vi "Main.vi"() -> ()   [LabVIEW 2015]
doc: "Use this template to build a simple state machine design pattern. Each state executes code and determines which state to transition to."
uses:
  controls/State.ctl
  controls/Data.ctl
panel:
  out "Current State":string
  out "Data":cluster{"X":dbl, "Y":dbl}[](graph)
  in  "Reset Settings":bool
  in  "Clear Graph":bool
  in  "Analyze Data":bool
  in  "Acquire Data":bool
  in  "Configure Data":bool
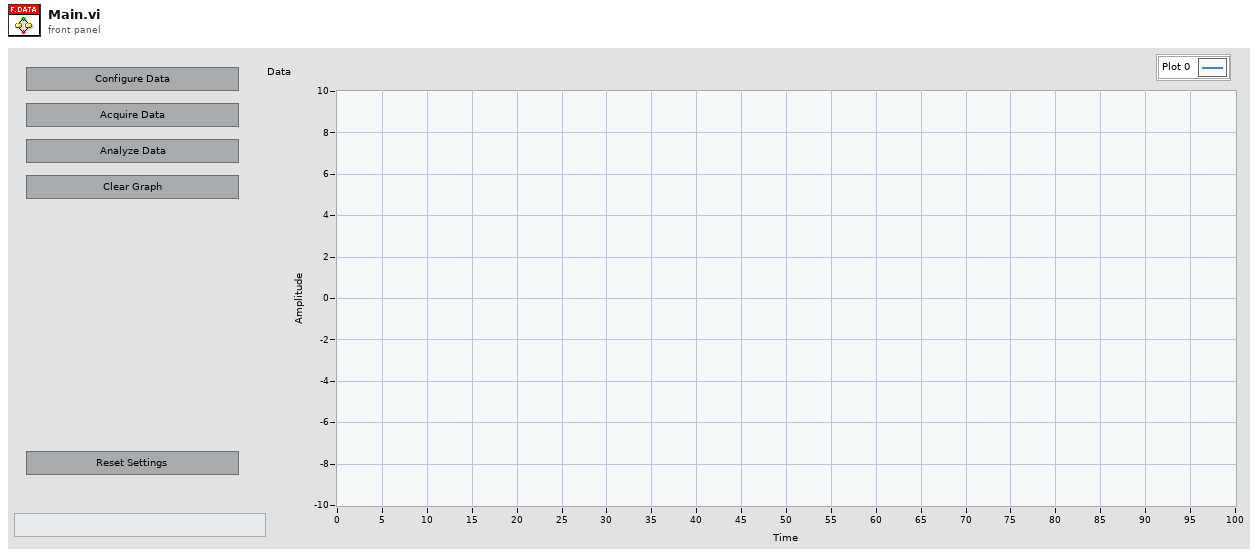
[diagram p1: front panel]
types:
  T1 = typedef "Data.ctl" = cluster{"Boolean <Replace Me>":bool, "String <Replace Me>":string, "Numeric <Replace Me>":dbl}
  T2 = typedef "State.ctl" = enum16{"Initialize", "Wait for Event", "Configure", "Acquire Data", "Update User Interface", "Reset Data", "Clear Data", "Analyse Data", "Stop", "Error"}
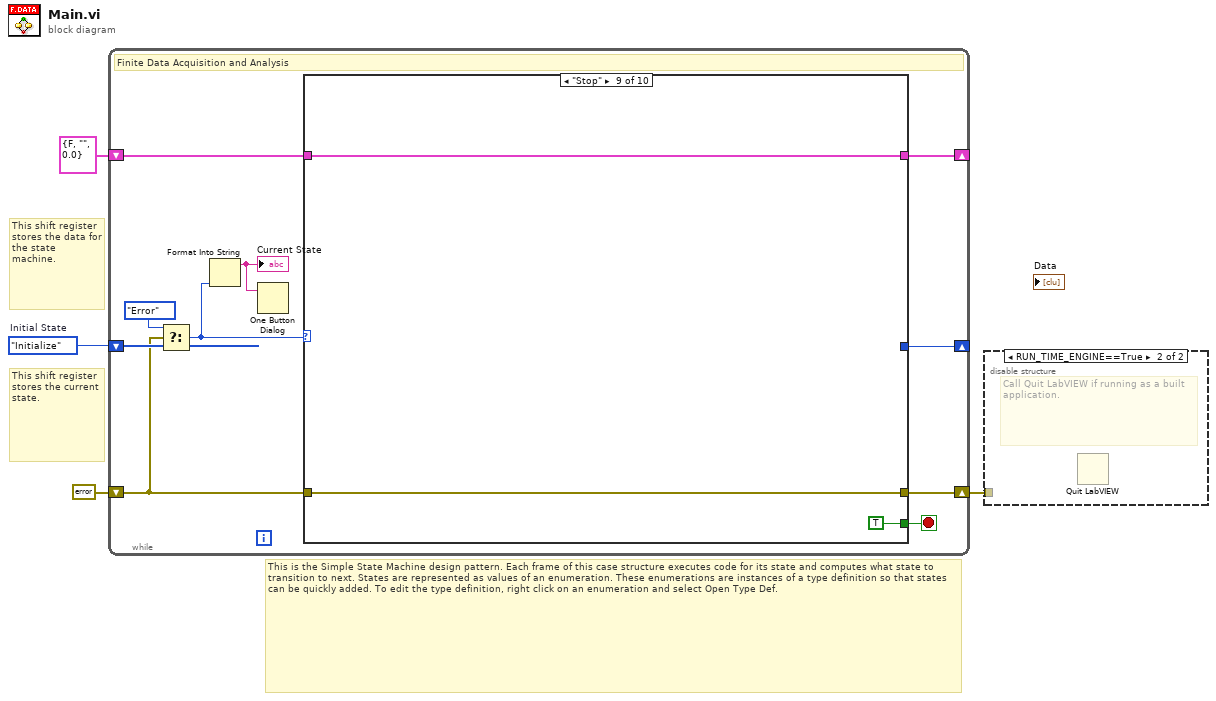
[diagram p0: block diagram]
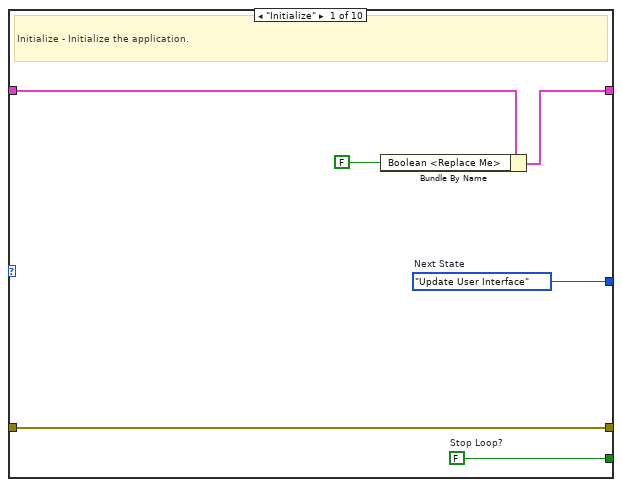
[diagram p3: hidden frame]
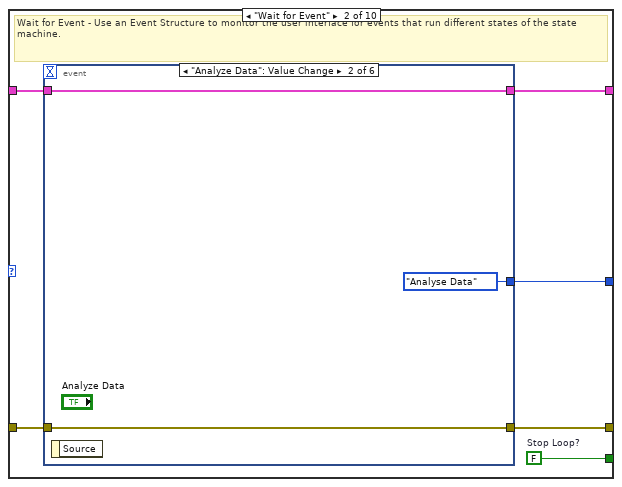
[diagram p4: hidden frame]
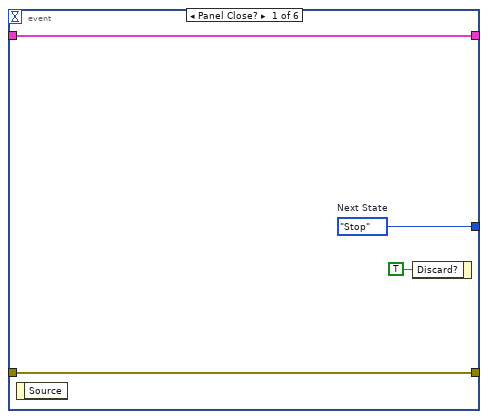
[diagram p5: hidden frame]
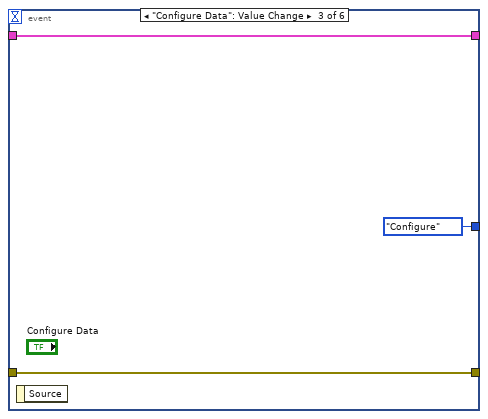
[diagram p6: hidden frame]
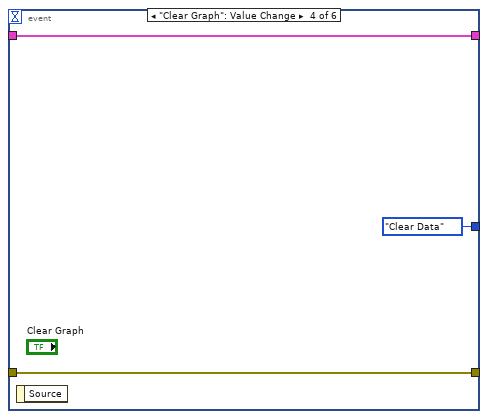
[diagram p7: hidden frame]
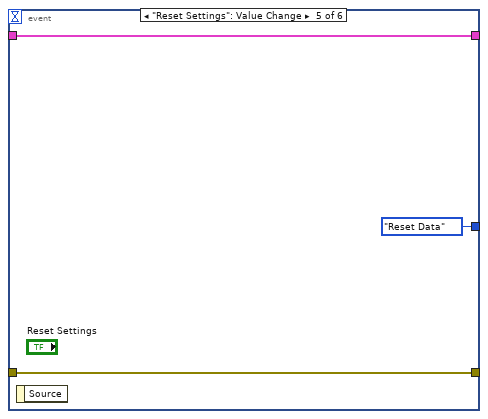
[diagram p8: hidden frame]
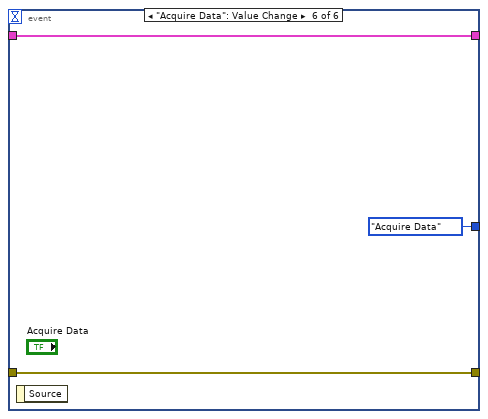
[diagram p9: hidden frame]
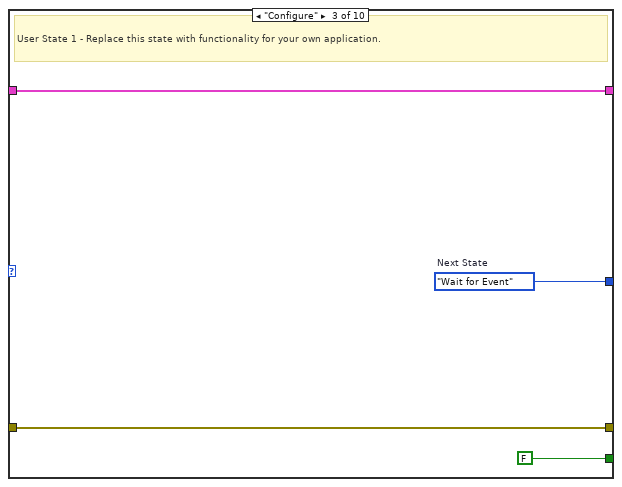
[diagram p10: hidden frame]
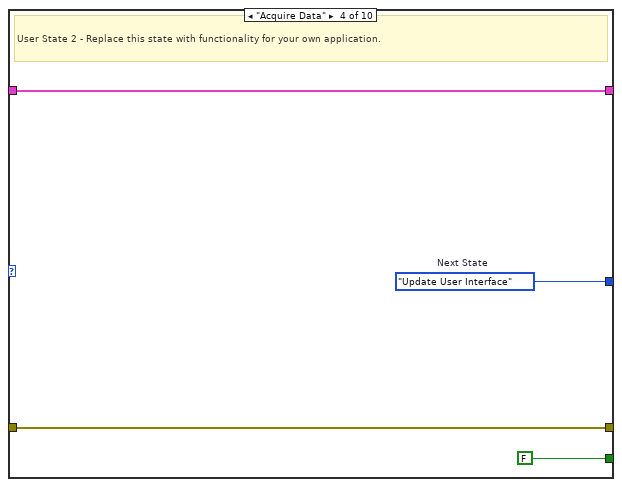
[diagram p11: hidden frame]
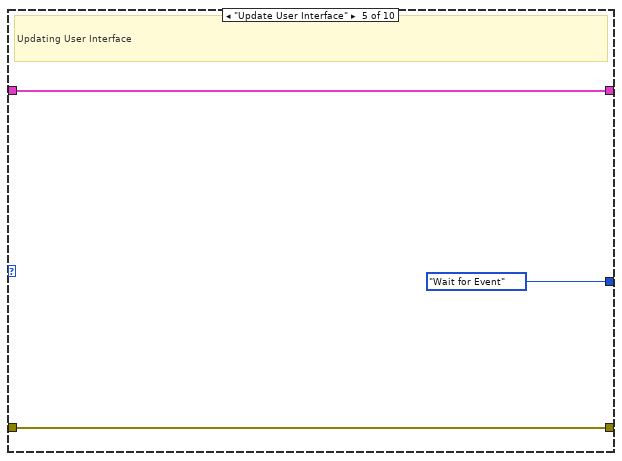
[diagram p12: hidden frame]
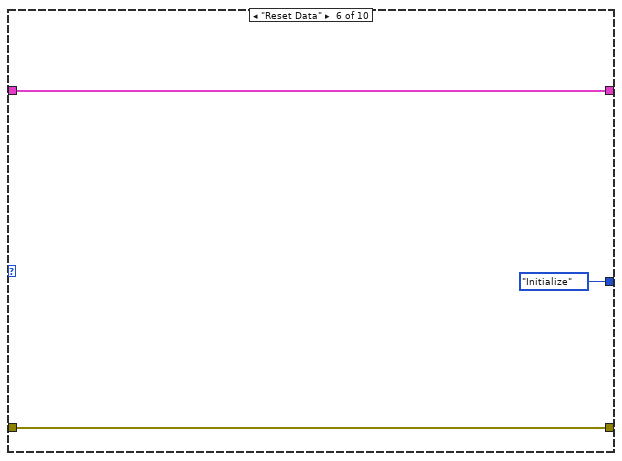
[diagram p13: hidden frame]
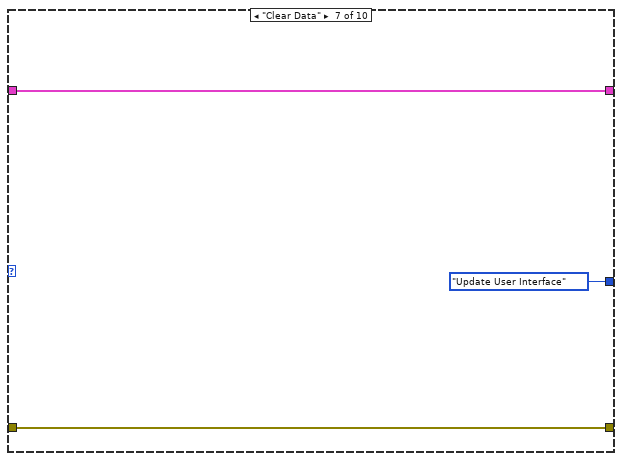
[diagram p14: hidden frame]
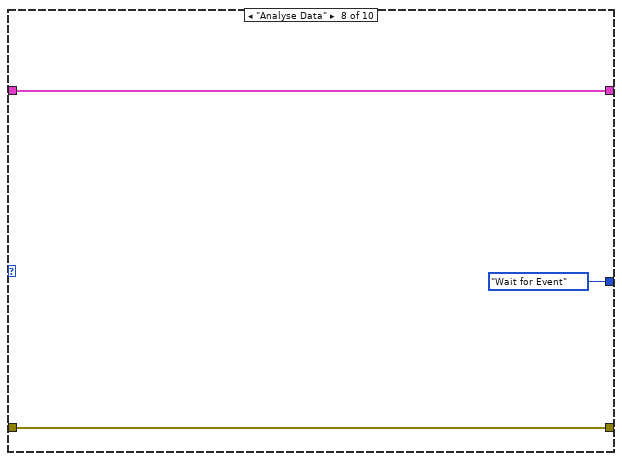
[diagram p15: hidden frame]
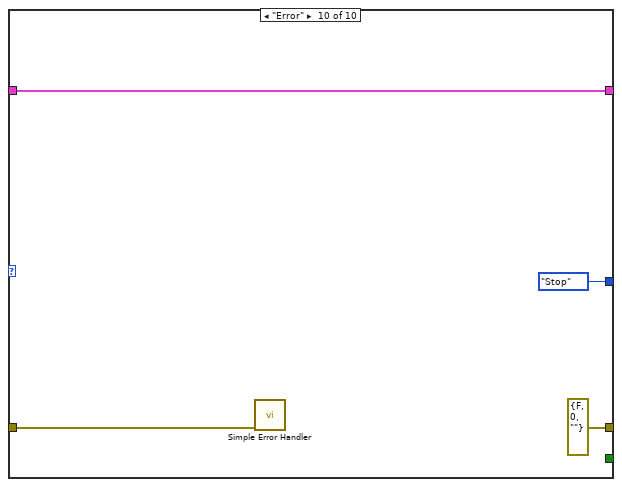
[diagram p16: hidden frame]
diagram:
  w4 = State."Initialize"  # Initial State
  # "This shift register stores the data for the state machine."
  # "This is the Simple State Machine design pattern. Each frame of this case structure executes code for its state and computes what state to transition to next. States are represented as values of an enumeration. These enumerations are instances of a type definition so that states can be quickly added. To edit the type definition, right click on an enumeration and select Open Type Def."
  # "This shift register stores the current state."
  n1 = while {
    shift-right: [w14] -> _
    shift-left: w4 -> [w9]
    shift-right: [w12] -> _
    shift-left: T1 {"Boolean <Replace Me>"=FALSE, "String <Replace Me>"="", "Numeric <Replace Me>"=0.0} ("Data") -> [w13]
    shift-right: [w11] -> w1
    shift-left: errorcluster {"status"=FALSE, "code"=0, "source"=""} ("error constant") -> [w10]
    stop <- w5 stop-if-true
    # "Finite Data Acquisition and Analysis"
    n2 = Select(t=State."Error", s=w10, f=w9) -> (s? t:f=w7:T2)
    n3 = Format Into String(w7) -> (resulting string=w6:string)  [unwired: 3 in, 1 out]
    "Current State" <- w6
    n4 = One Button Dialog(message=w6) -> ()  [unwired: 1 in, 1 out]
    n5 = case shown="\"Stop\"" w7 {
      tunnel: [w20 w26 w49 w53 State."Wait for Event" ("(Value Not Used)") State."Initialize" ("(Value Not Used)") State."Update User Interface" ("(Value Not Used)") State."Wait for Event" ("(Value Not Used)") _ State."Stop" ("(Value Not Used)")] -> w14
      tunnel: [w19 w25 FALSE ("Stop Loop?") FALSE ("Stop Loop?") _ _ _ _ TRUE ("Stop Loop?") _] -> w5
      tunnel: w13 -> [w18 w24 w47 w51 w55 w59 w62 w65 w68 w72]
      tunnel: [w17 w23 w47 w51 w55 w59 w62 w65 w68 w72] -> w12
      tunnel: w10 -> [w15 w22 w46 w50 w54 w58 w61 w64 w67 w70]
      tunnel: [w15 w21 w46 w50 w54 w58 w61 w64 w67 errorcluster {"status"=FALSE, "code"=0, "source"=""} ("error constant")] -> w11
      frame "Initialize" {
        w19 = FALSE  # Stop Loop?
        w20 = State."Update User Interface"  # Next State
        # "Initialize - Initialize the application."
        n6 = Bundle By Name(cluster=w18, "Boolean <Replace Me>"=FALSE ("Replace_Me_Boolean")) -> (w17:T1)
      }
      frame "Wait for Event" {
        w25 = FALSE  # Stop Loop?
        # "Wait for Event - Use an Event Structure to monitor the user interface for events that run different states of the state machine."
        n7 = event shown="[1] \"Analyze Data\": Value Change" {
          selector: _ -> [_ _ _ _ _ _]
          dyn-events: _ -> [_ _ _ _ _ _]
          timeout: _ -> [_ _ _ _ _ _]
          tunnel: [w30 State."Analyse Data" ("Next State") State."Configure" ("Next State") State."Clear Data" ("Next State") State."Reset Data" ("Next State") State."Acquire Data" ("Next State")] -> w26
          tunnel: w24 -> [w29 w33 w36 w39 w42 w45]
          tunnel: [w29 w33 w36 w39 w42 w45] -> w23
          tunnel: w22 -> [w28 w32 w35 w38 w41 w44]
          tunnel: [w28 w32 w35 w38 w41 w44] -> w21
          event Panel Close? {
            w30 = State."Stop"  # Next State
            n8 = event-data() -> ()  [unwired: 1 in, 1 out]
            n9 = event-data("Discard?"=TRUE) -> ()  [unwired: 1 in, 1 out]
          }
          event "Analyze Data": Value Change {
            n10 = event-data() -> ()  [unwired: 1 in, 1 out]
          }
          event "Configure Data": Value Change {
            n11 = event-data() -> ()  [unwired: 1 in, 1 out]
          }
          event "Clear Graph": Value Change {
            n12 = event-data() -> ()  [unwired: 1 in, 1 out]
          }
          event "Reset Settings": Value Change {
            n13 = event-data() -> ()  [unwired: 1 in, 1 out]
          }
          event "Acquire Data": Value Change {
            n14 = event-data() -> ()  [unwired: 1 in, 1 out]
          }
        }
      }
      frame "Configure" {
        w49 = State."Wait for Event"  # Next State
        # "User State 1 - Replace this state with functionality for your own application."
      }
      frame "Acquire Data" {
        w53 = State."Update User Interface"  # Next State
        # "User State 2 - Replace this state with functionality for your own application."
      }
      frame "Update User Interface" {
        # "Updating User Interface"
      }
      frame "Reset Data" {
      }
      frame "Clear Data" {
      }
      frame "Analyse Data" {
      }
      frame "Stop" {
      }
      frame "Error" {
        n15 = call <vilib>:"Simple Error Handler.vi"("error in (no error)"=w70) -> ()  [unwired: 4 in, 5 out]
      }
    }
  }
  n16 = disable-structure shown="RUN_TIME_ENGINE==True" {
    disable-tunnel: w1 -> [_ _]
    frame condition #0 (active) {
    }
    frame condition #1 {
      # "Call Quit LabVIEW if running as a built application."
      n17 = Quit LabVIEW() -> ()  [unwired: 1 in]
    }
  }
